vi "Write Header - Basic FITS info.vi"(8 "error in (no error)":errorcluster, 11 "Save Image in":refnum<class "Save Image.lvclass">) -> (0 "error out":errorcluster, 3 "Save Image out":refnum<class "Save Image.lvclass">)   [LabVIEW 2018, in "Save Image.lvclass"]
uses:
  Save Image.lvclass
  Simulated_Header/Simulated_Header.lvclass
  Interface/Interface.lvclass
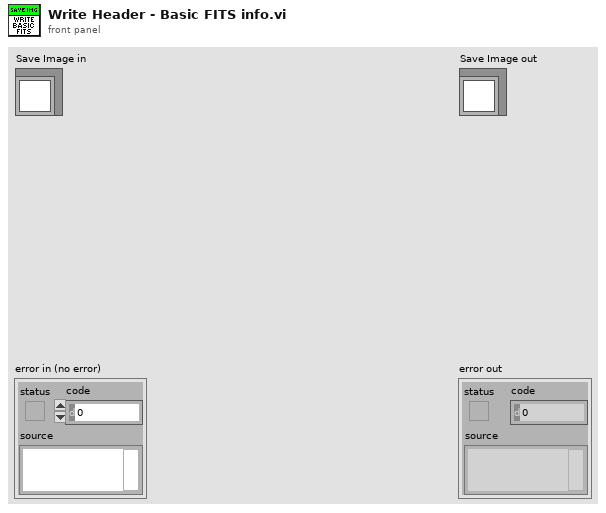
[diagram p1: front panel]
types:
  T1 = cluster{"COOLER_POWER_STATUS":u16, "TEMP":i32, "EXPTIME":sgl, "#FRAMES":u32, "#CUBES":u32}
  T2 = cluster{"PREAMP":u16, "READOUT_RATE":u16, "EM_GAIN":u16, "VBIN":u16, "INITIAL_LINE":u16, "INITIAL_COLUMN":u16, "FINAL_LINE":u16, "FINAL_COLUMN":u16, "TRIGGER_MODE":u16, "HBIN":u16, "SHUTTER_TTL":u16, "SHUTTER_MODE":u16, "SHUTTER_OPENING_TIME":u16, "SHUTTER_CLOSING_TIME":u16, "VERTICAL_SHIFT_SPEED":u16, "READ_MODE":u16, "FRAME_TRANSFER":bool, "VERTICAL_CLOCK_VOLTAGE":u16, "ACQUISITION_MODE":u16, "AD_CHANNEL":u16, "EM_MODE":u16}
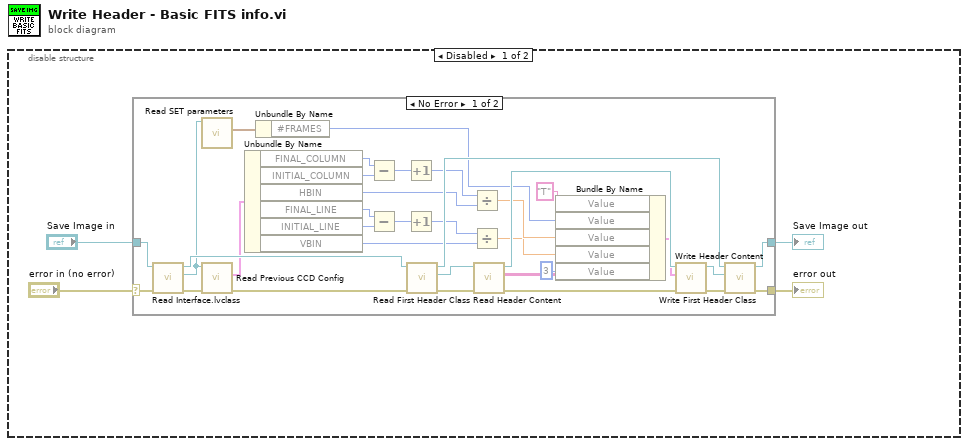
[diagram p0: block diagram]
diagram:
  n1 = disable-structure shown="Disabled" {
    frame Disabled {
      n2 = case shown="No Error" "error in (no error)" {
        selector: "error in (no error)" -> [w31 w39]
        tunnel: [w25 w39] -> w3
        tunnel: [w26 w40] -> w1
        tunnel: "Save Image in" -> [w30 w40]
        frame No Error {
          n3 = call "Read Interface.lvclass.vi"("error in (no error)"=w31, "Save Image in"=w30) -> ("error out"=w28:errorcluster, "Interface.lvclass"=w12:refnum<class "Interface.lvclass">, "Save Image out"=w29:refnum<class "Save Image.lvclass">)  [unwired: 7 in]
          n4 = call "Read SET parameters.vi"("Interface in"=w12) -> ("SET parameters"=w11:T1)  [unwired: 8 in, 2 out]
          n5 = call "Read Previous CCD Config.vi"("error in (no error)"=w28, "Interface in"=w12) -> ("error out"=w27:errorcluster, "CCD Config"=w14:T2)  [unwired: 7 in, 1 out]
          n6 = Unbundle By Name(w14) -> ("FINAL_COLUMN"=w24:u16, "INITIAL_COLUMN"=w23:u16, "HBIN"=w20:u16, "FINAL_LINE"=w22:u16, "INITIAL_LINE"=w21:u16, "VBIN"=w19:u16)
          n7 = Unbundle By Name(w11) -> ("#FRAMES"=w10:u32)
          n8 = Subtract(x=w24, y=w23) -> (x-y=w18:u16)
          n9 = Subtract(x=w22, y=w21) -> (x-y=w16:u16)
          n10 = Increment(x=w18) -> (x+1=w17:u16)
          n11 = Increment(x=w16) -> (x+1=w15:u16)
          n12 = call "Read First Header Class.vi"("error in (no error)"=w27, "Save Image in"=w29) -> ("error out"=w36:errorcluster, "Simulated_Header.lvclass"=w37:refnum<class "Simulated_Header.lvclass">, "Save Image out"=w38:refnum<class "Save Image.lvclass">)  [unwired: 7 in]
          n13 = Divide(x=w17, y=w20) -> (x/y=w9:dbl)
          n14 = Divide(x=w15, y=w19) -> (x/y=w8:dbl)
          n15 = call "Read Header Content.vi"("error in (no error)"=w36, "Simulated_Header in"=w37) -> ("error out"=w33:errorcluster, "Header Content"=w13:string[][], "Simulated_Header out"=w32:refnum<class "Simulated_Header.lvclass">)  [unwired: 7 in]
          n16 = Bundle By Name(cluster=w13, "Value"="T", "Value"=w10, "Value"=w9, "Value"=w8, "Value"=u32 3 ("NAXIS.Value")) -> (w7:cluster{})
          n17 = call "Write Header Content.vi"("error in (no error)"=w33, "Header Content"=w7, "Simulated_Header in"=w32) -> ("error out"=w34:errorcluster, "Simulated_Header out"=w35:refnum<class "Simulated_Header.lvclass">)  [unwired: 7 in]
          n18 = call "Write First Header Class.vi"("error in (no error)"=w34, "Simulated_Header.lvclass"=w35, "Save Image in"=w38) -> ("error out"=w25:errorcluster, "Save Image out"=w26:refnum<class "Save Image.lvclass">)  [unwired: 7 in]
        }
        frame Error {
        }
      }
      "error out" <- w3
      "Save Image out" <- w1
    }
    frame Enabled {
    }
  }
